vi "Check_Data_Quality.vi"(2 "Read sensor?":bool, 3 "Data in":sgl caption="Numeric") -> (0 "Display colour":u32(colorbox), 1 "Data out":dbl caption="Numeric")   [LabVIEW 2013]
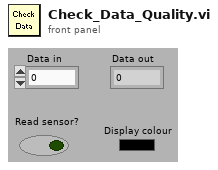
[diagram p1: front panel]
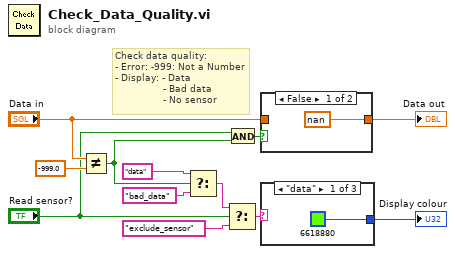
[diagram p0: block diagram]
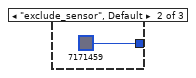
[diagram p3: hidden frame]
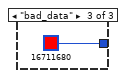
[diagram p4: hidden frame]
diagram:
  # "Check data quality:\n- Error: -999: Not a Number\n- Display: - Data\n                - Bad data\n                - No sensor"
  n1 = Not Equal?(x="Data in", y=sgl -999.0) -> (x != y?=w2:bool)
  n2 = Select(t="data", s=w2, f="bad_data") -> (s? t:f=w6:string)
  n3 = Select(t=w6, s="Read sensor?", f="exclude_sensor" ("t")) -> (s? t:f=w9:string)
  n4 = And(x="Read sensor?", y=w2) -> (x .and. y?=w1:bool)
  n5 = case shown="False" w1 {
    tunnel: "Data in" -> [_ w14]
    tunnel: [nan ("Data_input") w14] -> w8
    frame False {
    }
    frame True {
    }
  }
  "Data out" <- w8
  n6 = case shown="\"data\"" w9 {
    tunnel: [u32 6618880 u32 7171459 u32 16711680] -> w12
    frame "data" {
    }
    frame "exclude_sensor", Default {
    }
    frame "bad_data" {
    }
  }
  "Display colour" <- w12
